vi "COB send.vi"(4 "Data":u8[](array[numeric]), 5 "error in":errorcluster, 7 "COB id":i32, 8 "CANopen in":refnum<class "CANopen.lvclass">) -> (0 "error out":errorcluster, 3 "CANopen out":refnum<class "CANopen.lvclass">)   [LabVIEW 2024, in "canopen.lvlib" / "CANopen.lvclass"]
doc: "Sends a bunch of data to a specific COB-ID."
uses:
  CANopen.lvclass
  CANopen.lvclass/CANopen.ctl
  HAL/HAL/Protocols/ICAN/ICAN.lvclass
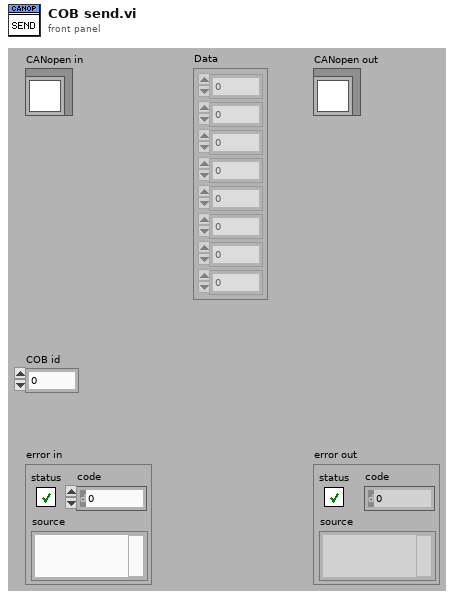
[diagram p1: front panel]
types:
  T1 = cluster{"ID":u32, "MSG type":u8, "DLC":u8, "DATA":u8[]}
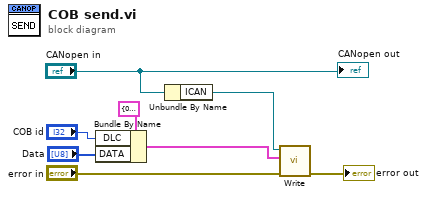
[diagram p0: block diagram]
diagram:
  n1 = Bundle By Name(cluster=T1 {"ID"=0, "MSG type"=0, "DLC"=0, "DATA"=[]} ("CAN Message"), "DLC"="COB id", "DATA"="Data") -> (w3:T1)
  n2 = Unbundle By Name("CANopen in") -> ("ICAN"=w2:refnum<class "ICAN.lvclass">)
  n3 = call-dynamic "Write.vi"("error in"="error in", "CAN Message"=w3, "ICAN in"=w2) -> ("error out"=→"error out":errorcluster)  [unwired: 7 in, 1 out]
  "CANopen out" <- "CANopen in"
